vi "Configure Waveform (Trapezoid).vi"(0 "VISA resource name":refnum<visa-resource-name>, 1 "Trapezoid Start Time (0.0 s)":dbl format="%^.3e", 2 "Trapezoid Start Level (0.0)":dbl format="%^.3e", 3 "Trapezoid Peak Width (1.0 s)":dbl=1.0 format="%^.3e", 5 "Channel Name (1)":string="1", 7 "Trapezoid Rise Time (1.0 s)":dbl=1.0 format="%^.3e", 9 "Waveform Type (1: Voltage)":i32(ring)=1 items=["Voltage"=1, "Current"=0], 11 "error in (no error)":errorcluster {"code" format="%.0x"}, 12 "Trapezoid End Time (0.0 s)":dbl format="%^.3e", 13 "Trapezoid Peak (0.0)":dbl format="%^.3e", 14 "Trapezoid Fall Time (1.0 s)":dbl=1.0 format="%^.3e") -> (4 "VISA resource name out":refnum<visa-resource-name>, 15 "error out":errorcluster {"code" format="%.0x"})   [LabVIEW 2018, in "Agilent N6700 Series.lvlib"]
doc: "Configures the trapezoid waveform.\n\n<b>Note:</b>\nThis VI only applies to the N6705B and N6705C DC Power Analyzer."
uses:
  Agilent N6700 Series.lvlib
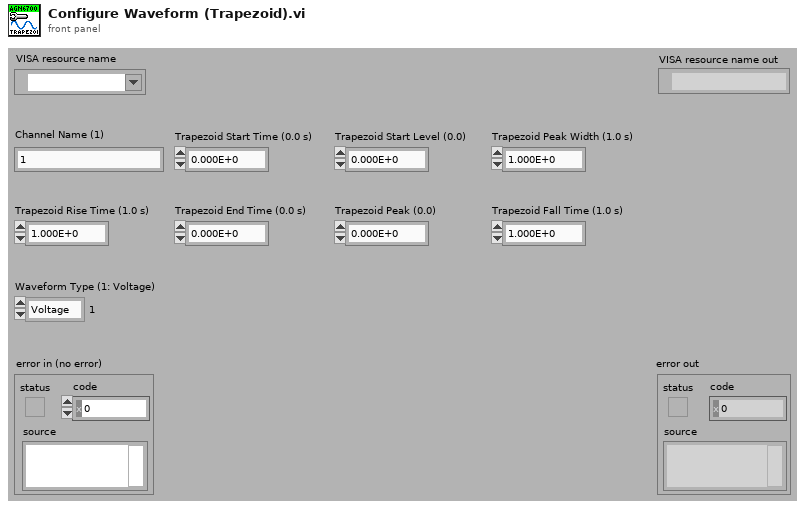
[diagram p1: front panel]
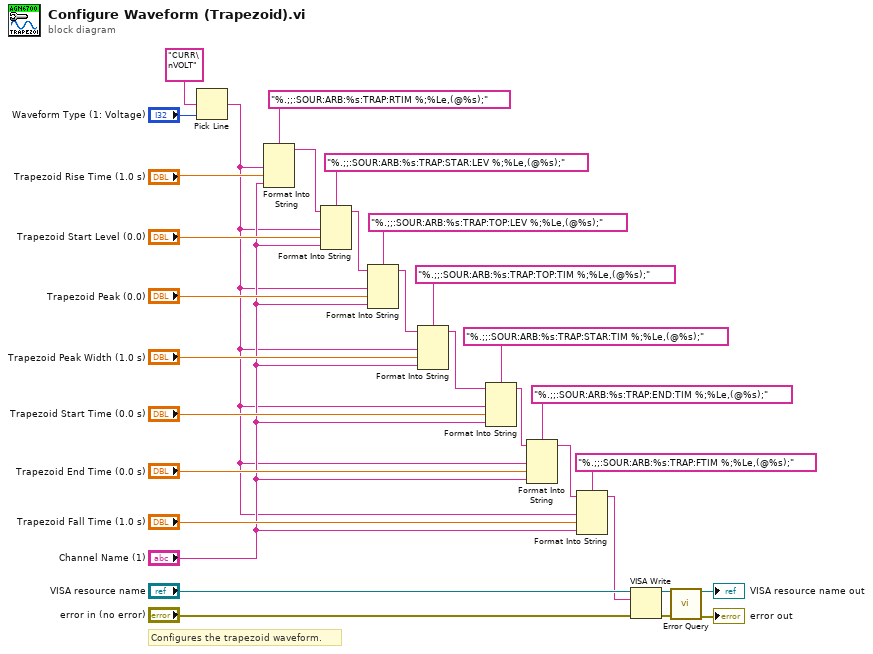
[diagram p0: block diagram]
diagram:
  # "Configures the trapezoid waveform."
  n1 = Pick Line(multi-line string="CURR\nVOLT", line index="Waveform Type (1: Voltage)") -> (output string=w1:string)  [unwired: 1 in]
  n2 = Format Into String(format string="%.;;:SOUR:ARB:%s:TRAP:RTIM %;%Le,(@%s);", w1, "Trapezoid Rise Time (1.0 s)", "Channel Name (1)") -> (resulting string=w3:string)  [unwired: 2 in, 1 out]
  n3 = Format Into String(format string="%.;;:SOUR:ARB:%s:TRAP:STAR:LEV %;%Le,(@%s);", initial string=w3, w1, "Trapezoid Start Level (0.0)", "Channel Name (1)") -> (resulting string=w21:string)  [unwired: 1 in, 1 out]
  n4 = Format Into String(format string="%.;;:SOUR:ARB:%s:TRAP:TOP:LEV %;%Le,(@%s);", initial string=w21, w1, "Trapezoid Peak (0.0)", "Channel Name (1)") -> (resulting string=w20:string)  [unwired: 1 in, 1 out]
  n5 = Format Into String(format string="%.;;:SOUR:ARB:%s:TRAP:TOP:TIM %;%Le,(@%s);", initial string=w20, w1, "Trapezoid Peak Width (1.0 s)", "Channel Name (1)") -> (resulting string=w19:string)  [unwired: 1 in, 1 out]
  n6 = Format Into String(format string="%.;;:SOUR:ARB:%s:TRAP:STAR:TIM %;%Le,(@%s);", initial string=w19, w1, "Trapezoid Start Time (0.0 s)", "Channel Name (1)") -> (resulting string=w18:string)  [unwired: 1 in, 1 out]
  n7 = Format Into String(format string="%.;;:SOUR:ARB:%s:TRAP:END:TIM %;%Le,(@%s);", initial string=w18, w1, "Trapezoid End Time (0.0 s)", "Channel Name (1)") -> (resulting string=w10:string)  [unwired: 1 in, 1 out]
  n8 = Format Into String(format string="%.;;:SOUR:ARB:%s:TRAP:FTIM %;%Le,(@%s);", initial string=w10, w1, "Trapezoid Fall Time (1.0 s)", "Channel Name (1)") -> (resulting string=w8:string)  [unwired: 1 in, 1 out]
  n9 = VISA Write(VISA resource name="VISA resource name", write buffer=w8, error in (no error)="error in (no error)") -> (VISA resource name out=w27:refnum<visa-resource-name>, error out=w26:errorcluster)  [unwired: 1 out]
  n10 = call "Error Query.vi"("VISA resource name"=w27, "error in (no error)"=w26) -> ("VISA resource name out"=→"VISA resource name out":refnum<visa-resource-name>, "error out"=→"error out":errorcluster)  [unwired: 10 in, 2 out]
